vi "writeToXML.vi"(8 "error in (no error)":errorcluster, 10 "ClassLabel":string, 11 "RotatorOffsetCommands in":refnum<class "RotatorOffsetCommands.lvclass">) -> (0 "error out":errorcluster, 2 "XML out":string, 3 "RotatorOffsetCommands out":refnum<class "RotatorOffsetCommands.lvclass">)   [LabVIEW 2014, in "TCSDataDefinitions.lvlib" / "TCSCommand.lvlib" / "OffsetCommands.lvlib" / "RotatorOffsetCommands.lvclass"]
uses:
  RotatorOffsetCommands.lvclass
  OffsetCommands/OffsetCommands.lvclass
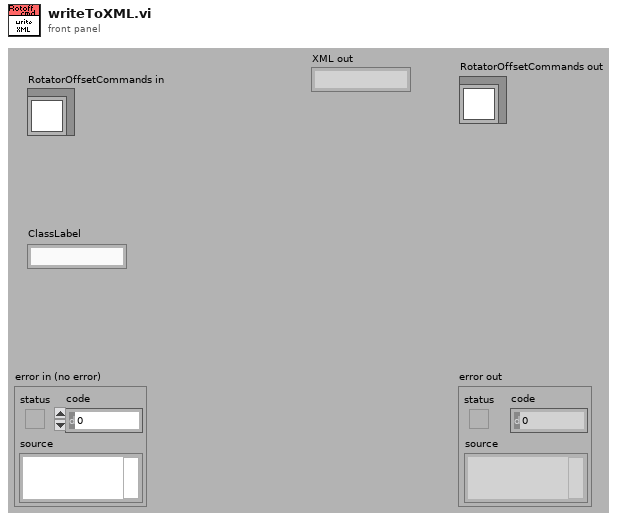
[diagram p1: front panel]
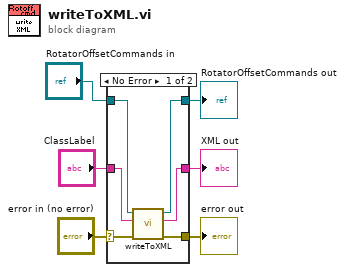
[diagram p0: block diagram]
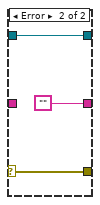
[diagram p2: hidden frame]
diagram:
  n1 = case shown="No Error" "error in (no error)" {
    selector: "error in (no error)" -> [w9 w15]
    tunnel: [w8 w15] -> w5
    tunnel: [w10 w14] -> w4
    tunnel: "RotatorOffsetCommands in" -> [w11 w14]
    tunnel: "ClassLabel" -> [w12 _]
    tunnel: [w7 ""] -> w2
    frame No Error {
      n2 = call-parent "writeToXML.vi"("error in (no error)"=w9, "ClassLabel"=w12, "OffsetCommands in"=w11) -> ("error out"=w8:errorcluster, "XML out"=w7:string, "OffsetCommands out"=w10:refnum<class "RotatorOffsetCommands.lvclass">)  [unwired: 6 in]
    }
    frame Error {
    }
  }
  "error out" <- w5
  "RotatorOffsetCommands out" <- w4
  "XML out" <- w2
